vi "FPGA Additive Timer.vi"(11 "Numeric in":u32) -> (3 "Numeric out":u32)   [LabVIEW 2014]
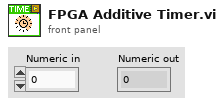
[diagram p1: front panel]
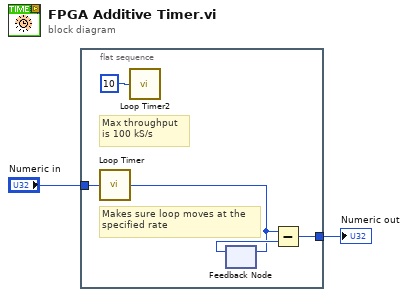
[diagram p0: block diagram]
diagram:
  n1 = flat-sequence {
    tunnel: "Numeric in" -> [w7]
    tunnel: [w4] -> w2
    frame #0 {
      # "Max throughput\nis 100 kS/s"
      # "Makes sure loop moves at the\nspecified rate"
      n2 = call "Loop Timer"("Count(Ticks)"=w7) -> ("Tick Count(Ticks)"=w5:u32)
      n3 = call "Loop Timer2"("Count(uSec)"=u8 10 ("Count(Ticks)")) -> ()  [unwired: 1 out]
      n4 = feedback-in #1(w5) -> ()
      n5 = feedback #1() -> (w6:u32)  [unwired: 1 out]
      n6 = Subtract(x=w5, y=w6) -> (x-y=w4:u32)
    }
  }
  "Numeric out" <- w2
